vi "PicoScope4000ExampleRapidBlock.vi"() -> ()   [LabVIEW 2012]
doc: "This example demonstrates how to use the PicoScope Labview library to collect data using rapid block mode, retrieving the data values in bulk."
uses:
  shared/PicoBuffers.ctl
  shared/Segment Range.ctl
  shared/Acquisition Settings.ctl
  shared/nSegments.ctl
  PicoScope4000Lib/PicoScope4000AnalogChannelSettingsIEPE.ctl
  PicoScope4000Lib/PicoScope4000Buffer and Transfer Settings.ctl
panel:
  out "Analog Channels (Min)":cluster{i32, dbl, "Data":dbl[]}[](graph)
  in  "Channel B Settings":T1={"Enabled"=TRUE, "Range"=6, "Bandwidth Limit"=0, "Coupling"=1} {"Coupling" items=["AC", "DC", "IEPE"]; "Bandwidth Limit" items=["Off", "200kHz"]; "Range" items=["10 mV", "20 mV", "50 mV", "100 mV", "200 mV", "500 mV", "1 V", "2 V", "5 V", "10 V", "20 V", "50 V ", "100 V"]}
  in  "Buffer and Transfer Settings":T2={"startIndex"=0, "Samples"=1000000, "Down Sample Ratio"=10, "Down-Sample Mode"=1} {"Down-Sample Mode" items=["None", "Aggregate", "Average"]; "Down Sample Ratio" step=1; "Samples" format="%_6p"}
  out "Overflow":i16[](array[numeric]) format="%04b"
  in  "Trigger Settings":T3={"Trigger Enabled"=FALSE, "Trigger Source"=enum."Channel A", "Trigger Threshold (Volts)"=0.0, "Trigger Direction"=2, "Trigger Delay (samples)"=0, "Auto Trigger Time (ms)"=1000} {"Trigger Direction" items=["Rising"=2, "Falling"=3]}
  out "nCaptures":u64=10 format="%.4p"
  in  "Channel A Settings":T1={"Enabled"=TRUE, "Range"=6, "Bandwidth Limit"=0, "Coupling"=1} {"Coupling" items=["AC", "DC", "IEPE"]; "Bandwidth Limit" items=["Off", "200kHz"]; "Range" items=["10 mV", "20 mV", "50 mV", "100 mV", "200 mV", "500 mV", "1 V", "2 V", "5 V", "10 V", "20 V", "50 V ", "100 V"]}
  in  "PicoScope 4262 Ext. Trigger Range":u32(ring)=5 items=["500 mV"=5, "5 V"=8]
  out "Unit Info":T4
  in  "Stop Display":bool
  out "Capture Complete":bool=TRUE
  in  "Run":bool
  in  "Display Buffer Index":i32
  in  "Segment Range":T5={"fromSegmentIndex"=0, "toSegmentIndex"=9} {"toSegmentIndex" format="%.4p"; "fromSegmentIndex" format="%.4p"}
  in  "nSegments":T6=10 format="%.4p"
  out "error out":errorcluster
  in  "Data file":path=path "PicoScope4000ExampleRapidBlock ChA Data"
  in  "Acquisition Settings":T7={"preTriggerSamples"=0, "postTriggerSamples"=1000000, "timebase"=5} {"postTriggerSamples" format="%_6p"; "preTriggerSamples" format="%_6p"}
  out "Properties Panel":T8 {"Max Total Capture Time Available (sec)" format="%.3p"; "Sample Frequency" format="%.6p"; "Sample Rate" format="%.3p"; "Max Samples Available" format="%_6p"; "Total Capture Time (sec)" format="%.3p"}
  in  "stop":bool
  out "Analog Channels":cluster{i32, dbl, "Data":dbl[]}[](graph)
  in  "Serial Number":string
  in  "Use Serial Number":bool
  in  "error in (no error)":errorcluster
  # "Number of\nSegments to Capture"
  # "Bit 0 = ChA"
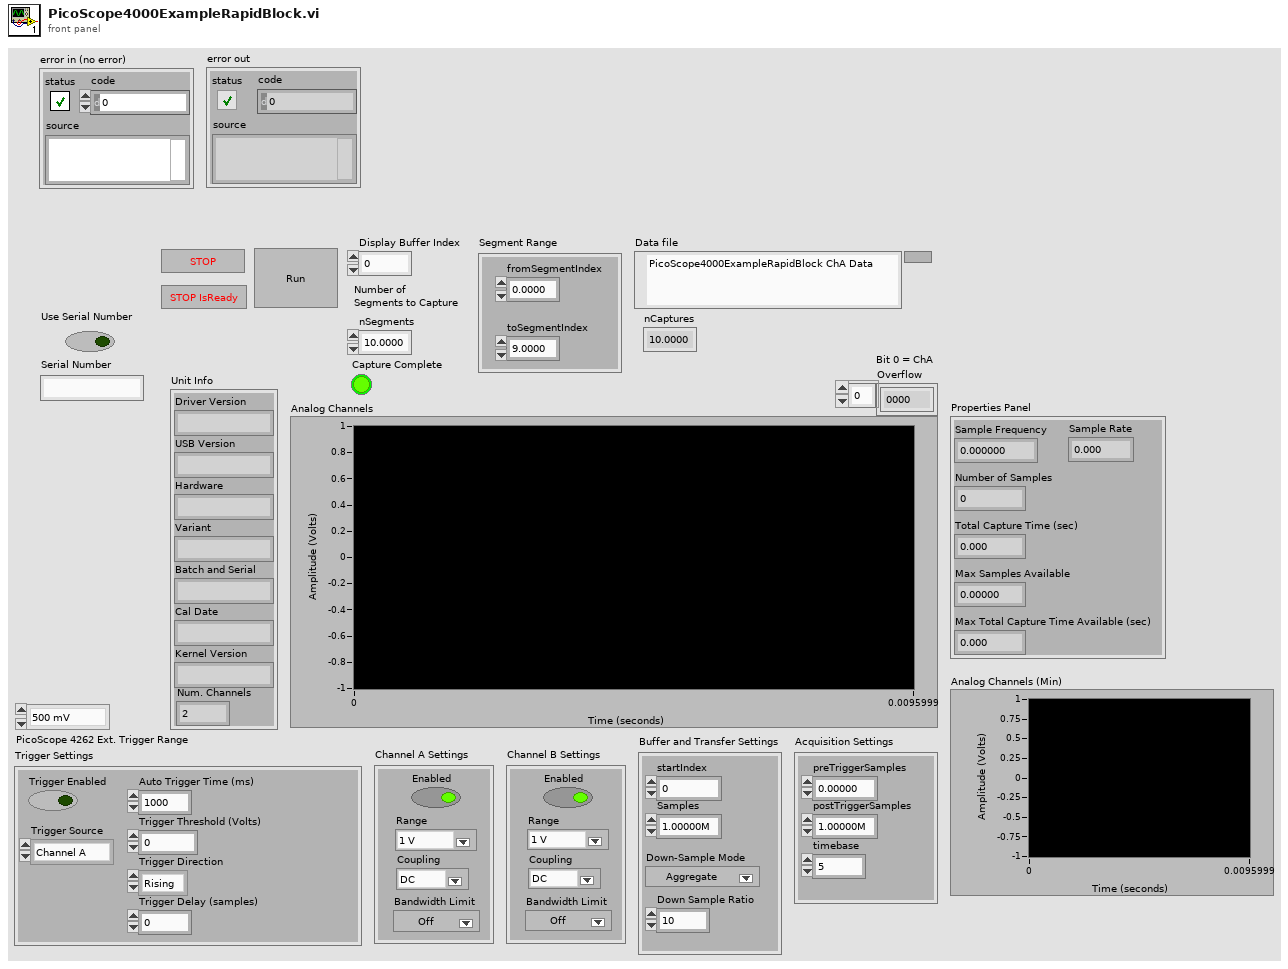
[diagram p1: front panel]
types:
  T1 = typedef "PicoScope4000AnalogChannelSettingsIEPE.ctl" = cluster{"Enabled":bool, "Range":u16, "Bandwidth Limit":i16, "Coupling":u16}
  T2 = typedef "PicoScope4000Buffer and Transfer Settings.ctl" = cluster{"startIndex":u64, "Samples":u64, "Down Sample Ratio":u64, "Down-Sample Mode":u32}
  T3 = cluster{"Trigger Enabled":bool, "Trigger Source":enum16{"Channel A", "Channel B", "Channel C", "Channel D", "Channel E", "Channel F", "Channel G", "Channel H"}, "Trigger Threshold (Volts)":dbl, "Trigger Direction":u16, "Trigger Delay (samples)":u32, "Auto Trigger Time (ms)":i16}
  T4 = cluster{"Driver Version":string, "USB Version":string, "Hardware":string, "Variant":string, "Batch and Serial":string, "Cal Date":string, "Kernel Version":string, "Num. Channels":i16}
  T5 = typedef "Segment Range.ctl" = cluster{"fromSegmentIndex":u64, "toSegmentIndex":u64}
  T6 = typedef "nSegments.ctl" = u64
  T7 = typedef "Acquisition Settings.ctl" = cluster{"preTriggerSamples":u64, "postTriggerSamples":u64, "timebase":u32}
  T8 = cluster{"Sample Frequency":dbl, "Sample Rate":dbl, "Max Samples Available":u64, "Number of Samples":u64, "Total Capture Time (sec) ":dbl, "Max Total Capture Time Available (sec)":dbl}
  T9 = enum16{"open", "open or create", "create or replace", "create", "open (read-only)"}
  T10 = typedef "PicoBuffers.ctl" = cluster{"Max Buffer Pointers":u64[][][], "Min Buffer Pointers":u64[][][], "StreamingDataInfo":cluster{"Channel":u32, "Down-Sample Mode":u32, "PICO_DATA_TYPE":enum32{"PICO_INT8_T", "PICO_INT16_T", "PICO_INT32_T", "PICO_UINT32_T", "PICO_INT64_T", ""}, "Samples":i32, "bufferIndex":u64, "startIndex":i32, "overflow":i16}[][]}
  T11 = cluster{"Channel A Buffer":i16[], "Channel B Buffer":i16[], "Channel C Buffer":i16[], "Channel D Buffer":i16[], "Channel E Buffer":i16[], "Channel F Buffer":i16[], "Channel G Buffer":i16[], "Channel H Buffer":i16[], "Port 0 Buffer":i16[], "Port 1 Buffer":i16[]}[]
  T12 = cluster{"Channel A Buffer":i16[], "Channel B Buffer":i16[], "Channel C Buffer":i16[], "Channel D Buffer":i16[], "Channel E Buffer":i16[], "Channel F Buffer":i16[], "Channel G Buffer":i16[], "Channel H Buffer":i16[], "Port 0 Buffer":i16[], "Port 1 Buffer":i16[]}
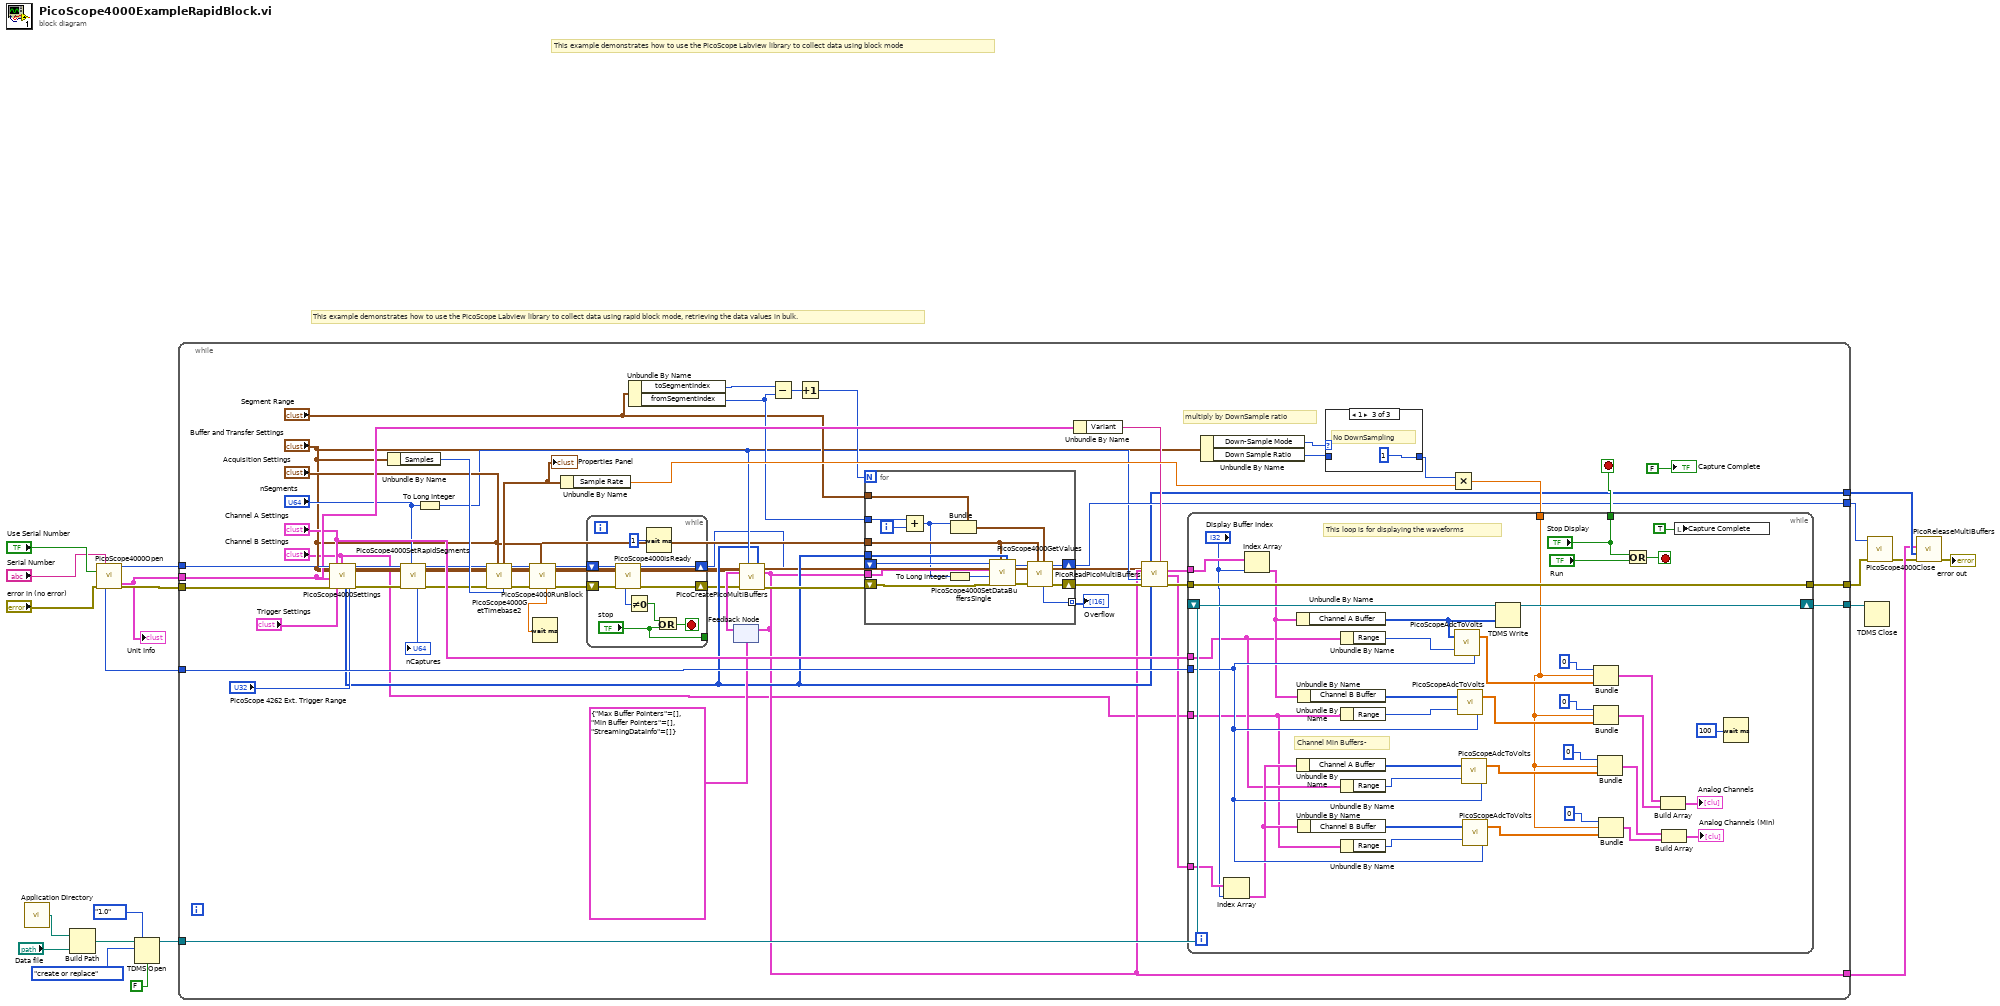
[diagram p0: block diagram]
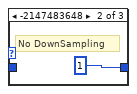
[diagram p3: hidden frame]
diagram:
  # "This example demonstrates how to use the PicoScope Labview library to collect data using rapid block mode, retrieving the data values in bulk."
  # "This example demonstrates how to use the PicoScope Labview library to collect data using block mode"
  n1 = call <vilib>:"Application Directory.vi"() -> ("Application Directory"=w15:path)
  n2 = Build Path(base path=w15, name or relative path="Data file") -> (appended path=w16:path)
  n3 = call "PicoScope4000Open.vi"("Serial Number"="Serial Number", "Use Serial Number"="Use Serial Number", "error in (no error)"="error in (no error)") -> ("handle"=w11:i16, "Max ADC value"=w12:i16, "Unit Info"=w6:T4, "error out"=w7:errorcluster)  [unwired: 9 in]
  "Unit Info" <- w6
  n4 = TDMS Open(6:FALSE ("disable buffering? (T)"), 7:enum16{"1.0", "2.0"}."1.0" ("file format version (2.0)"), 10:T9."create or replace" ("operation (0:open)"), 11:w16) -> (3:w13:refnum<k34>)  [unwired: 2 in, 1 out]
  n5 = while {
    tunnel: w12 -> [w61]
    tunnel: [w36] -> w21
    tunnel: [w30] -> w3
    tunnel: [w74] -> w14
    tunnel: w13 -> [w73]
    tunnel: w11 -> [w63]
    tunnel: [w62] -> w5
    tunnel: w7 -> [w55]
    tunnel: w6 -> [w51]
    tunnel: [w29] -> w2
    stop <- w65 stop-if-true
    # "multiply by DownSample ratio"
    n6 = call "PicoScope4000Settings.vi"("handle in"=w63, "Unit Info"=w51, "error in"=w55, "Channel A Settings"="Channel A Settings", "Trigger Settings"="Trigger Settings", "Channel B Settings"="Channel B Settings", "PicoScope 4262 Ext. Trigger Range"="PicoScope 4262 Ext. Trigger Range") -> ("Enabled array"=w30:i16[], "handle out"=w54:i16, "error out"=w53:errorcluster)  [unwired: 10 in]
    n7 = Unbundle By Name("Buffer and Transfer Settings") -> ("Samples"=w47:u64)
    n8 = call "PicoScope4000SetRapidSegments.vi"("nSegments"="nSegments", "error in (no error)"=w53, "handle in"=w54) -> ("error out"=w27:errorcluster, "handle out"=w26:i16, "nCaptures"=→"nCaptures":u64)  [unwired: 6 in]
    n9 = To Long Integer(number="nSegments") -> (32bit integer=w33:i32)
    n10 = call "PicoScope4000GetTimebase2.vi"("Number of Samples"=w47, "Acquisition Settings"="Acquisition Settings", "error in (no error)"=w27, "handle in"=w26) -> ("error out"=w57:errorcluster, "handle out"=w58:i16, "Properties Panel"=w69:T8)  [unwired: 5 in]
    "Properties Panel" <- w69
    n11 = call "PicoScope4000RunBlock.vi"("Acquisition Settings"="Acquisition Settings", "error in (no error)"=w57, "handle in"=w58) -> ("error out"=w37:errorcluster, "handle out"=w38:i16, "timeIndisposedMs"=w56:dbl)  [unwired: 5 in, 1 out]
    n12 = Wait (ms)(milliseconds to wait=w56) -> ()  [unwired: 1 out]
    n13 = Unbundle By Name(w69) -> ("Sample Rate"=w60:dbl)
    n14 = while {
      shift-right: [w137] -> w24
      shift-left: w37 -> [w138]
      shift-right: [w136] -> w23
      shift-left: w38 -> [w135]
      tunnel: ["stop"] -> _
      stop <- w132 stop-if-true
      n15 = call "PicoScope4000IsReady.vi"("error in (no error)"=w138, "handle in"=w135) -> ("error out"=w137:errorcluster, "handle out"=w136:i16, "ready"=w134:i16)  [unwired: 7 in]
      n16 = Not Equal To 0?(x=w134) -> (x != 0?=w133:bool)
      n17 = Wait (ms)(milliseconds to wait=u32 1) -> ()  [unwired: 1 out]
      n18 = Or(x=w133, y="stop") -> (x .or. y?=w132:bool)
    }
    n19 = Unbundle By Name("Segment Range") -> ("toSegmentIndex"=w44:u64, "fromSegmentIndex"=w43:u64)
    n20 = feedback #1(T10 {"Max Buffer Pointers"=[], "Min Buffer Pointers"=[], "StreamingDataInfo"=[]} ("Data Pointers")) -> (w32:T10)
    n21 = call "PicoCreatePicoMultiBuffers.vi"("Number of Buffers"=w33, "Buffer and Transfer Settings"="Buffer and Transfer Settings", "enabled array"=w30, "Data Pointers In"=w32, "error in (no error)"=w24) -> ("Data Pointers"=w29:T10, "error out"=w34:errorcluster)  [unwired: 9 in]
    n22 = feedback-in #1(w29) -> ()
    n23 = Subtract(x=w44, y=w43) -> (x-y=w41:u64)
    n24 = Increment(x=w41) -> (x+1=w40:u64)
    n25 = for {
      N: w40 -> [_]
      shift-right: [w90] -> w36
      shift-left: w23 -> [w81]
      shift-right: [w89] -> w35
      shift-left: w34 -> [w82]
      tunnel: w43 -> [w76]
      tunnel: "Segment Range" -> [w87]
      tunnel: [w85] -> w42 mode=indexing
      tunnel: w29 -> [w80]
      tunnel: w30 -> [w79]
      tunnel: "Buffer and Transfer Settings" -> [w78]
      i -> [w88]
      n26 = Add(x=w76, y=w88) -> (x+y=w75:u64)
      n27 = To Long Integer(number=w75) -> (32bit integer=w77:i32)
      n28 = Bundle(cluster=w87, "fromSegmentIndex"=w75) -> (w86:T5)  [unwired: 1 in]
      n29 = call "PicoScope4000SetDataBuffersSingle.vi"("enabled array"=w79, "Buffer and Transfer Settings"=w78, "error in (no error)"=w82, "waveform"=w77, "Data Pointers In"=w80, "handle in"=w81) -> ("error out"=w84:errorcluster, "handle out"=w83:i16)  [unwired: 4 in]
      n30 = call "PicoScope4000GetValues.vi"("Segment Range"=w86, "Buffer and Transfer Settings"=w78, "error in (no error)"=w84, "handle in"=w83) -> ("error out"=w89:errorcluster, "handle out"=w90:i16, "overflow"=w85:i16)  [unwired: 4 in, 1 out]
    }
    "Overflow" <- w42
    n31 = Unbundle By Name(w51) -> ("Variant"=w59:string)
    n32 = call "PicoReadPicoMultiBuffers.vi"("enabled array"=w30, "Buffer and Transfer Settings"="Buffer and Transfer Settings", "Variant"=w59, "Data Pointers"=w29, "No of Buffers"=w33, "error in (no error)"=w35) -> ("MultiBuffers (Max or non-aggregated)"=w72:T11, "Min Buffers"=w28:T11, "error out"=w66:errorcluster)  [unwired: 7 in]
    n33 = Unbundle By Name("Buffer and Transfer Settings") -> ("Down-Sample Mode"=w70:u32, "Down Sample Ratio"=w71:u64)
    n34 = case shown="1" w70 {
      tunnel: [w139 u64 1 ("Down Sample Ratio") u64 1 ("Down Sample Ratio")] -> w67
      tunnel: w71 -> [w139 _ _]
      frame Default {
      }
      frame -2147483648 {
        # "No DownSampling"
      }
      frame 1 {
        # "No DownSampling"
      }
    }
    n35 = Multiply(x=w67, y=w60) -> (x*y=w68:dbl)
    n36 = while {
      tunnel: w61 -> [w104]
      tunnel: "Channel A Settings" -> [w92]
      tunnel: w72 -> [w112]
      tunnel: w68 -> [w105]
      shift-right: [w129] -> w74
      shift-left: w73 -> [w128]
      tunnel: [w118] -> w62
      tunnel: w66 -> [w118]
      tunnel: ["Stop Display"] -> w65
      tunnel: w28 -> [w103]
      tunnel: "Channel B Settings" -> [w91]
      stop <- w115 stop-if-true
      # "Channel Min Buffers-"
      # "This loop is for displaying the waveforms"
      n37 = Index Array(array=w103, index="Display Buffer Index") -> (element=w101:T12)
      n38 = Index Array(array=w112, index="Display Buffer Index") -> (element=w100:T12)
      n39 = Unbundle By Name(w100) -> ("Channel A Buffer"=w119:i16[])
      n40 = Unbundle By Name(w101) -> ("Channel A Buffer"=w110:i16[])
      n41 = Unbundle By Name(w100) -> ("Channel B Buffer"=w125:i16[])
      n42 = Unbundle By Name(w101) -> ("Channel B Buffer"=w107:i16[])
      n43 = Unbundle By Name(w92) -> ("Range"=w95:u16)
      n44 = Unbundle By Name(w91) -> ("Range"=w96:u16)
      n45 = Unbundle By Name(w92) -> ("Range"=w94:u16)
      n46 = Unbundle By Name(w91) -> ("Range"=w93:u16)
      n47 = call "PicoScopeAdcToVolts.vi"("Max_adc"=w104, "Range Index"=w95, "Data"=w119) -> ("Data"=w120:dbl[])
      n48 = call "PicoScopeAdcToVolts.vi"("Max_adc"=w104, "Range Index"=w96, "Data"=w125) -> ("Data"=w124:dbl[])
      n49 = call "PicoScopeAdcToVolts.vi"("Max_adc"=w104, "Range Index"=w94, "Data"=w110) -> ("Data"=w109:dbl[])
      n50 = call "PicoScopeAdcToVolts.vi"("Max_adc"=w104, "Range Index"=w93, "Data"=w107) -> ("Data"=w106:dbl[])
      n51 = TDMS Write(0:w128, 9:w119) -> (4:w129:refnum<k34>)  [unwired: 4 in, 3 out]
      n52 = Bundle(0, w105, "Data"=w120) -> (w123:cluster{i32, dbl, "Data":dbl[]})  [unwired: 1 in]
      n53 = Bundle(0, w105, "Data"=w124) -> (w122:cluster{i32, dbl, "Data":dbl[]})  [unwired: 1 in]
      n54 = Bundle(0, w105, "Data"=w109) -> (w98:cluster{i32, dbl, "Data":dbl[]})  [unwired: 1 in]
      n55 = Bundle(0, w105, "Data"=w106) -> (w97:cluster{i32, dbl, "Data":dbl[]})  [unwired: 1 in]
      n56 = Or(x="Stop Display", y="Run") -> (x .or. y?=w115:bool)
      n57 = Build Array(w123, w122) -> (→"Analog Channels":cluster{i32, dbl, "Data":dbl[]}[])
      n58 = Build Array(w98, w97) -> (→"Analog Channels (Min)":cluster{i32, dbl, "Data":dbl[]}[])
      n59 = local write "Capture Complete"(TRUE ("Capture Complete")) -> ()
      n60 = Wait (ms)(milliseconds to wait=u32 100) -> ()  [unwired: 1 out]
    }
    "Capture Complete" <- FALSE ("Capture Complete")
  }
  n61 = TDMS Close(11:w14) -> ()  [unwired: 1 in, 2 out]
  n62 = call "PicoScope4000Close.vi"("error in (no error)"=w5, "handle"=w21) -> ("error out"=w1:errorcluster)  [unwired: 9 in]
  n63 = call "PicoReleaseMultiBuffers.vi"("error in (no error)"=w1, "Enabled array"=w3, "Data Pointers"=w2) -> ("error out"=→"error out":errorcluster)  [unwired: 8 in]
